vi "initialise_keithley.vi"(10 "Scan settings":T1={"Start voltage (V)"=0.0, "End voltage (V)"=1.4, "Number of steps"=10, "Measurement delay (ms)"=10.0, "Dual sweep"=0, "Stabilisation time (s)"=0.0, "Stabilisation mode"=0, "Stabilisation value (V or A) "=0.0, "No. of repeat scans"=2.0, "Repeat scans"=0, "Logarithmic sweep"=0, "Electrode configuration"=0} {"Electrode configuration" items=["2-wire", "4-wire"]; "Logarithmic sweep" items=["False", "True"]; "Repeat scans" items=["False", "True"]; "No. of repeat scans" min=1.0 step=1.0; "Stabilisation mode" items=["V", "I"]; "Dual sweep" items=["False", "True"]; "Measurement delay (ms)" min=10.0}, 11 "VISA Refnum in":refnum<visa-resource-name>="GPIB1::26::INSTR") -> (0 "error out":errorcluster, 3 "VISA Refnum out":refnum<visa-resource-name>)   [LabVIEW 2016]
uses:
  TypeDefs/settings.ctl
  TypeDefs/nplc_for_j-v_scan.ctl
  <instrlib>/Keithley 24XX/Keithley 24XX.lvlib
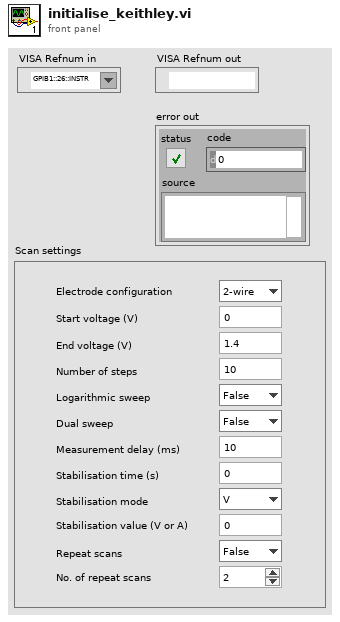
[diagram p1: front panel]
types:
  T1 = typedef "settings.ctl" = cluster{"Start voltage (V)":dbl, "End voltage (V)":dbl, "Number of steps":u32, "Measurement delay (ms)":dbl, "Dual sweep":u16, "Stabilisation time (s)":dbl, "Stabilisation mode":u16, "Stabilisation value (V or A) ":dbl, "No. of repeat scans":dbl, "Repeat scans":u16, "Logarithmic sweep":u16, "Electrode configuration":u16}
  T2 = typedef "nplc_for_j-v_scan.ctl" = dbl
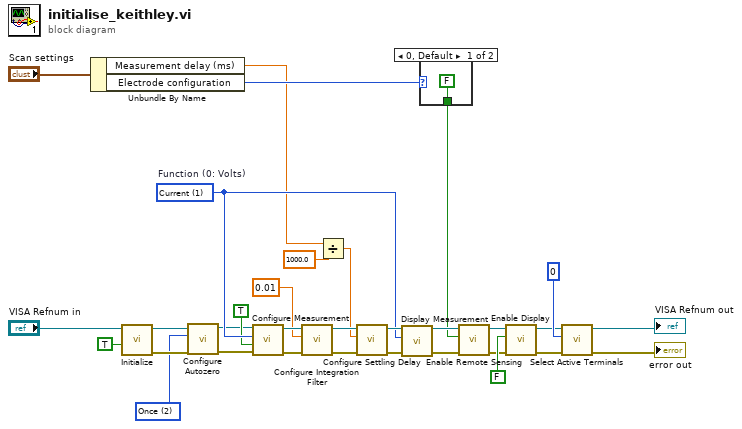
[diagram p0: block diagram]
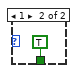
[diagram p2: hidden frame]
diagram:
  w5 = u16 2 items=["On", "Off", "Once"] ("Autozero  (0: On)")
  w17 = u16 1 items=["Volts", "Current", "Resistance"]  # Function (0: Volts)
  n1 = Unbundle By Name("Scan settings") -> ("Measurement delay (ms)"=w2:dbl, "Electrode configuration"=w3:u16)
  n2 = call <instrlib>:"Initialize.vi"("Reset (True)"=TRUE, "VISA resource name"="VISA Refnum in") -> ("error out"=w8:errorcluster, "VISA resource name out"=w9:refnum<visa-resource-name>)  [unwired: 3 in, 5 out]
  n3 = call <instrlib>:"Configure Autozero.vi"("error in (no error)"=w8, "Autozero  (0: On)"=w5, "VISA resource name"=w9) -> ("error out"=w6:errorcluster, "VISA resource name out"=w7:refnum<visa-resource-name>)  [unwired: 7 in]
  n4 = call <instrlib>:"Configure Measurement.vi"("error in (no error)"=w6, "Enable Auto Range (T:Enable)"=TRUE, "Function (0: Volts)"=w17, "VISA resource name"=w7) -> ("error out"=w22:errorcluster, "VISA resource name out"=w23:refnum<visa-resource-name>)  [unwired: 6 in]
  n5 = call <instrlib>:"Configure Integration Filter.vi"("error in (no error)"=w22, "Measurement Speed (1 PLC)"=T2 0.01, "VISA resource name"=w23) -> ("error out"=w15:errorcluster, "VISA resource name out"=w16:refnum<visa-resource-name>)  [unwired: 7 in]
  n6 = Divide(x=w2, y=1000.0) -> (x/y=w11:dbl)
  n7 = call <instrlib>:"Configure Settling Delay.vi"("error in (no error)"=w15, "Manual Settling Delay (0 sec)"=w11, "VISA resource name"=w16) -> ("error out"=w18:errorcluster, "VISA resource name out"=w19:refnum<visa-resource-name>)  [unwired: 7 in]
  n8 = call <instrlib>:"Display Measurement.vi"("error in (no error)"=w18, "Displayed Measurement (0: Voltage)"=w17, "VISA resource name"=w19) -> ("error out"=w20:errorcluster, "VISA resource name out"=w21:refnum<visa-resource-name>)  [unwired: 7 in]
  n9 = case shown="0, Default" w3 {
    tunnel: [FALSE ("Enable Output (T: Enable)") TRUE ("Enable Output (T: Enable)")] -> w1
    frame 0, Default {
    }
    frame 1 {
    }
  }
  n10 = call <instrlib>:"Enable Remote Sensing.vi"("error in (no error)"=w20, "Enable Remote Sensing (T: Enable)"=w1, "VISA resource name"=w21) -> ("error out"=w25:errorcluster, "VISA resource name out"=w24:refnum<visa-resource-name>)  [unwired: 7 in]
  n11 = call <instrlib>:"Enable Display.vi"("error in (no error)"=w25, "Enable Display (T: Enable)"=FALSE, "VISA resource name"=w24) -> ("error out"=w27:errorcluster, "VISA resource name out"=w26:refnum<visa-resource-name>)  [unwired: 7 in]
  n12 = call <instrlib>:"Select Active Terminals.vi"("error in (no error)"=w27, "Active Terminals (0: Front)"=0, "VISA resource name"=w26) -> ("error out"=→"error out":errorcluster, "VISA resource name out"=→"VISA Refnum out":refnum<visa-resource-name>)  [unwired: 7 in]
